vi "FTW-JSON-Object-Keys.vi"(0 "JSON Object":refnum<class "FTW-JSON.lvclass">, 11 "error in":errorcluster) -> (4 "JSON Object out":refnum<class "FTW-JSON.lvclass">, 6 "Keys":string[](array[string]), 15 "error out":errorcluster)   [LabVIEW 2015, in "FTW-JSON.lvclass"]
uses:
  FTW-JSON.lvclass
  FTW-JSON.lvclass/FTW-JSON.ctl
panel:
  # "Inputs"
  # "Outputs"
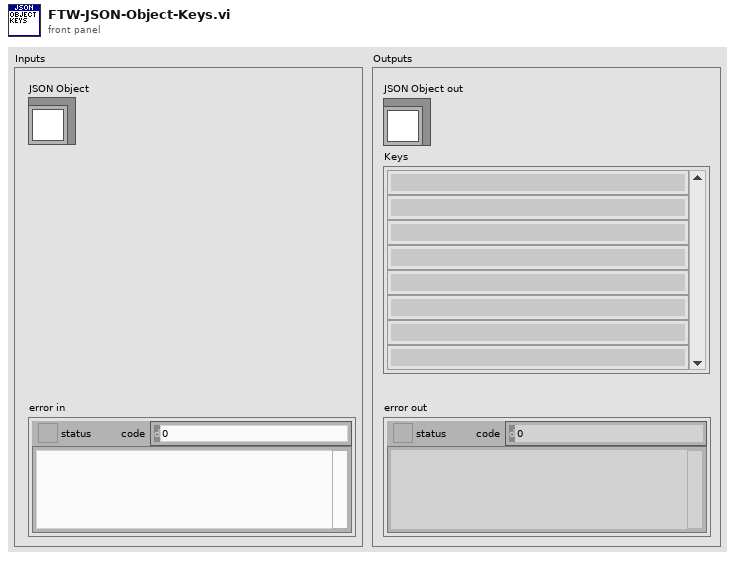
[diagram p1: front panel]
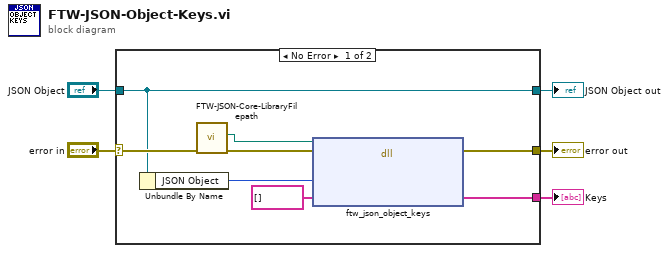
[diagram p0: block diagram]
diagram:
  n1 = case shown="No Error" "error in" {
    selector: "error in" -> [w13 w15]
    tunnel: [w6 w15] -> w5
    tunnel: [w12 w14] -> w3
    tunnel: "JSON Object" -> [w12 w14]
    tunnel: [w7 _] -> w1
    frame No Error {
      n2 = Unbundle By Name(w12) -> ("JSON Object"=w9:i64)
      n3 = call "FTW-JSON-Core-LibraryFilepath.vi"("error in"=w13) -> ("error out"=w11:errorcluster, "JSON Library Filepath"=w10:path)  [unwired: 9 in]
      n4 = dll-call lib="?" fn="ftw_json_object_keys"(path in=w10, error in=w11, "JSON Object Pointer"=w9, "Keys"=string[] []) -> (error out=w6:errorcluster, "Keys"=w7:string[])  [unwired: 3 in, 1 out]
    }
    frame Error {
    }
  }
  "error out" <- w5
  "JSON Object out" <- w3
  "Keys" <- w1
